vi "Top Level FPGA_w8LED.vi"() -> ()   [LabVIEW 2012]
uses:
  <vilib>/Platform/TimedLoop/XDataNode/timing_clust.ctl
  <vilib>/Platform/TimedLoop/XDataNode/nitl_modes.ctl
  <vilib>/Platform/TimedLoop/XDataNode/wakeup.ctl
  <vilib>/rvi/DataTransferAndStorage/Container/Common/niFpgaContainerMetaDataKey.ctl
  <vilib>/rvi/DataTransferAndStorage/Container/Common/niFpgaContainerState.ctl
  <vilib>/rvi/DataTransferAndStorage/Container/Common/niFpgaDataTypeControl.ctl
  <vilib>/rvi/DataTransferAndStorage/Container/Common/niFpgaContainerImplementationControl.ctl
  <vilib>/rvi/DataTransferAndStorage/Container/Common/niFpgaContainerArbitrationOptionsControl.ctl
  <vilib>/rvi/DataTransferAndStorage/Container/Common/niFpgaTransferTypeControl.ctl
  <vilib>/rvi/DataTransferAndStorage/Container/Common/niFpgaContainerInitializationParameters.ctl
  <vilib>/rvi/Memory/Memory_Types/niFpgaMemoryInterfaceConfiguration.ctl
  <vilib>/rvi/FIFO/Fifo_Types/niFpgaFifoControlLogicControl.ctl
  <vilib>/rvi/eio/common/nirviEmuTemplateMethod_errors.vi
  <vilib>/rvi/FIFO/Fifo_Resource/nirvififoEmulationSetSize.vi
  <vilib>/rvi/DataTransferAndStorage/Container/Common/niFpgaContainerGetUniqueNameForEmu.vi
  <vilib>/rvi/Emulation/niFpgaSctlEmulationRegisterWithScheduler.vi
  <vilib>/rvi/Emulation/niFpgaSctlEmulationScheduler.vi
  <vilib>/rvi/DataTransferAndStorage/Container/Common/niFpgaContainerSetEmuInfo.vi
  <vilib>/rvi/eio/common/nirviEmuReportErrorAndStop.vi
  <vilib>/rvi/Emulation/niFpgaSctlEmulationFifoFullMgr.vi
  <vilib>/rvi/errors/niFpgaSetErrorForExecOnDevCompSimple.vi
  <vilib>/rvi/Memory/Memory_Emulation/nirvimemoryEmulationManagerCache_GetValue.vi
  <vilib>/rvi/Memory/Memory_Emulation/niFpgaMemoryEmulationValidateCache.vi
  <vilib>/rvi/Memory/Memory_Emulation/nirvimemoryEmulationManagerCache_InsertValue.vi
  <vilib>/rvi/Memory/Memory_Emulation/nirvimemoryEmulationManagerCache_SetValue.vi
  <vilib>/rvi/Emulation/niFpgaSctlEmulationResourceMgr.vi
  <vilib>/rvi/Memory/Memory_Emulation/niFpgaMemoryEmulationCacheClearOnFirstRun.vi
  <vilib>/rvi/Memory/Memory_Emulation/nirvimemoryEmulationManagerCache_MakeExclusive.vi
  <vilib>/rvi/Memory/Memory_Emulation/nirvimemoryEmulationManagerCache_ReleaseExclusive.vi
  <vilib>/Utility/error.llb/Clear Errors.vi
  <vilib>/eio/EIONode/EIONode.xnode
  <vilib>/Platform/TimedLoop/XDataNode/XDataNode.xnode
  <vilib>/rvi/DataTransferAndStorage/Container/XNode/niFpgaContainer.xnode
  <vilib>/rvi/FIFO/Fifo_Resource/nirvififoEmulationClear.vi
  <vilib>/rvi/LocalResourceManager/LocalResourceManager.xnode
  <vilib>/rvi/FIFO/Fifo_Resource/nirvififoEmulationRead.vi
  <vilib>/rvi/DataTransferAndStorage/Register/Emulation/niFpgaRegisterEmulation.vi
  <vilib>/rvi/Memory/Memory_Emulation/nirvimemoryEmulation.vi
  <vilib>/rvi/FIFO/Fifo_Resource/nirvififoEmulationWrite.vi
  <vilib>/Platform/TimedLoop/XDataNode/XDNodeRunTimeDep.lvlib
panel:
  out "IO Module\\ADC Error A":bool
  out "IO Module\\ADC Error B":bool
  out "IO Module\\Pll Unlocked":bool
  in  "Record Size only data":u32=95
  out "DMA FIFO Timed Out?":bool
  in  "circular buffer length":u32=1000
  in  "location":i16(ring) items=["Purdue", "NIKHEF", "Zurich", "???"]
  in  "Trigger 0":i16=4000
  in  "Trigger 1":i16=4000
  in  "Trigger 2":i16=4000
  in  "Trigger 3":i16=4000
  in  "Trigger 4":i16=4000
  in  "Trigger 5":i16=4000
  in  "Trigger 6":i16=4000
  in  "Trigger 7":i16=4000
  in  "# of pretrigger":u32=20
  in  "initial value":u64
  in  "channel 0 on/off":bool
  in  "channel 2 on/off":bool
  in  "channel 1 on/off":bool
  in  "channel 3 on/off":bool
  in  "channel 4 on/off":bool
  in  "channel 5 on/off":bool
  in  "channel 6 on/off":bool
  in  "channel 7 on/off":bool
  in  "Testpulse duration (20 ns ticks)":u32=1
  in  "Testpulse Separation (20 ns ticks)":u32=500
  in  "Testpulse Time Delay (20 ns ticks)":u32=15
  out "Timestamp":u64
  in  "Testpulser On/Off":bool
  out "Init Done":bool
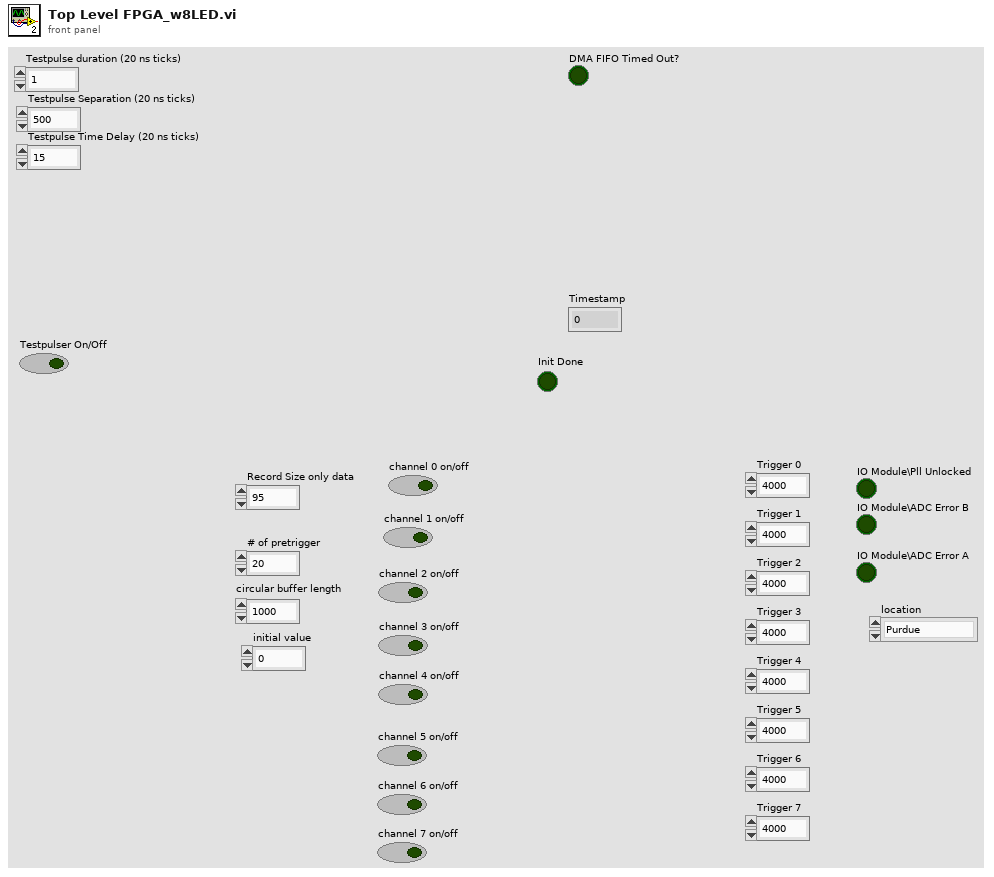
[diagram p1: front panel]
types:
  T1 = typedef "XDNodeRunTimeDep.lvlib/timing_clust.ctl" = cluster{"Expected End [f-1]":u64, "Actual End [f-1]":u64, "Finished Late? [f-1]":bool, "Expected End [i-1]":u64, "Actual End [i-1]":u64, "Finished Late? [i-1]":bool, "Expected Start [i]":u64, "Actual Start [i]":u64, "Expected Start [f]":u64, "Actual Start [f]":u64, "Source Name":string, "Structure Name":string, "Period":i64, "Deadline":i64, "Offset":i64, "Start":i64, "Priority":i32, "Timeout":i32, "Mode":T2, "Wakeup Reason":T3, "Error":errorcluster, "Source Type":string, "Secondary Source Type":string, "Global End Time":u64, "Global Start Time":u64, "Frame Duration":u64, "Iteration Duration":u64, "Assigned CPU":i32, "I/O Scan Engine Mode":u32}
  T2 = typedef "XDNodeRunTimeDep.lvlib/nitl_modes.ctl" = enum32{"No Change", "Process missed periods, maintain original phase", "Discard missed periods, maintain original phase", "Process missed periods, ignore original phase", "Discard missed periods, ignore original phase"}
  T3 = typedef "XDNodeRunTimeDep.lvlib/wakeup.ctl" = enum32{"Normal", "Aborted", "Asynchronous wakeup", "Timing source error", "Timed loop error", "Timeout"}
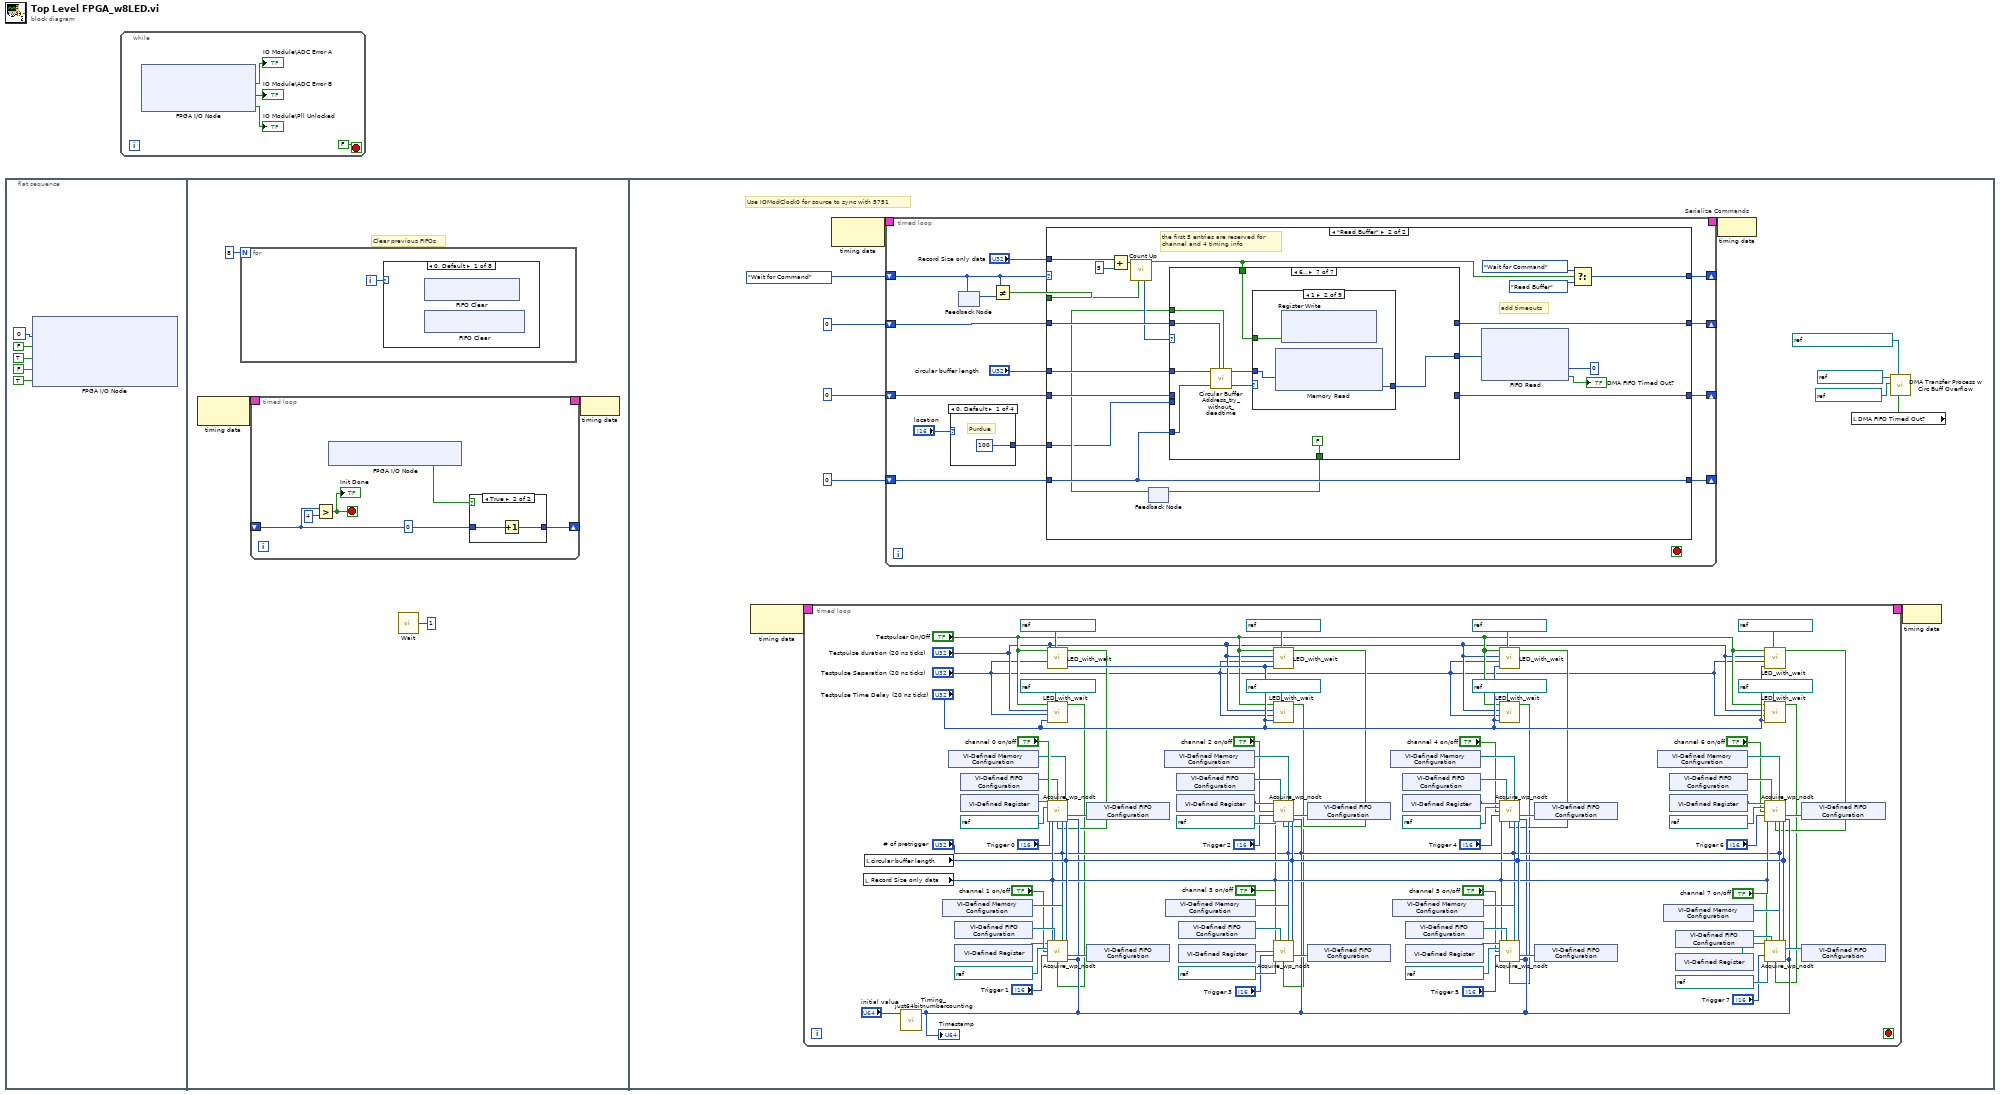
[diagram p0: block diagram]
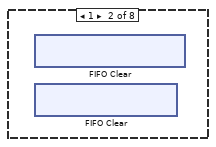
[diagram p2: hidden frame]
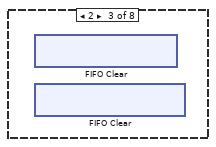
[diagram p3: hidden frame]
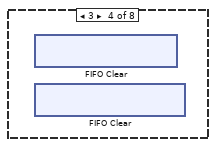
[diagram p4: hidden frame]
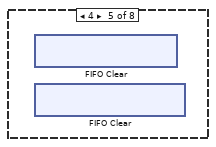
[diagram p5: hidden frame]
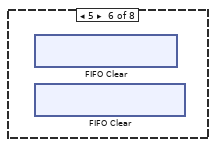
[diagram p6: hidden frame]
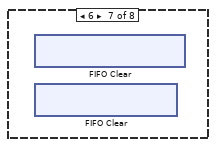
[diagram p7: hidden frame]
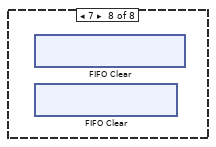
[diagram p8: hidden frame]
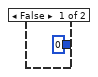
[diagram p9: hidden frame]
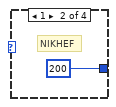
[diagram p10: hidden frame]
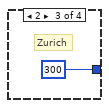
[diagram p11: hidden frame]
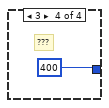
[diagram p12: hidden frame]
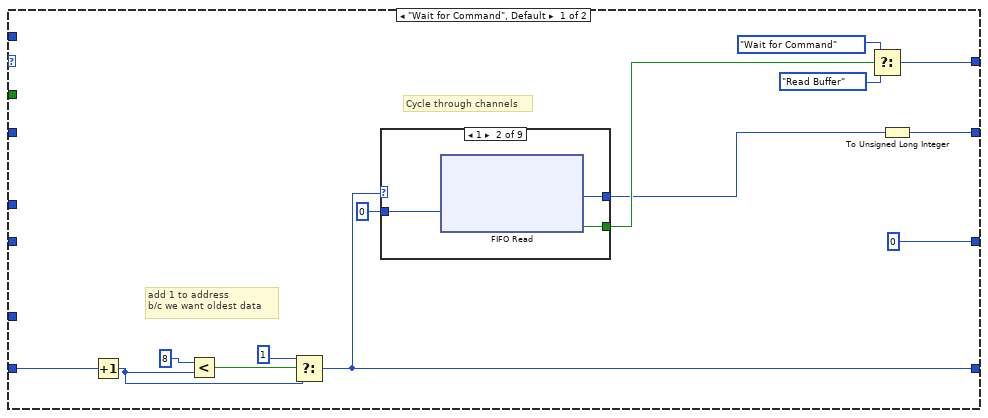
[diagram p13: hidden frame]
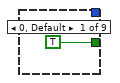
[diagram p14: hidden frame]
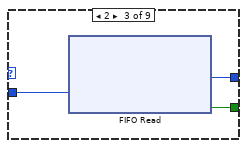
[diagram p15: hidden frame]
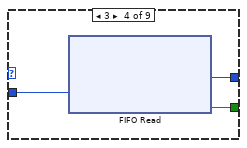
[diagram p16: hidden frame]
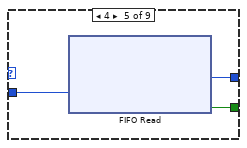
[diagram p17: hidden frame]
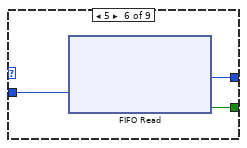
[diagram p18: hidden frame]
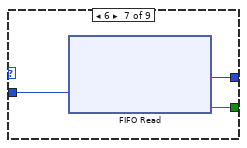
[diagram p19: hidden frame]
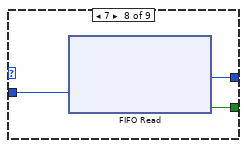
[diagram p20: hidden frame]
diagram:
  n1 = flat-sequence {
    frame #0 {
      n2 = xnode "FPGA I/O Node"("IO Module\\Sample Clock Select"=u8 0 ("IO Module\\Sample Clock Select"), "IO Module\\Force Initialization"=FALSE ("IO Module\\Force Initialization"), "IO Module\\Force Initialization"=TRUE ("IO Module\\Force Initialization"), "IO Module\\Force Initialization"=FALSE ("IO Module\\Force Initialization"), "IO Module\\Digital Output Enable"=TRUE ("IO Module\\Digital Output Enable")) -> ()  [unwired: 5 in, 5 out]
    }
    frame #1 {
      # "Clear previous FIFOs"
      n3 = node-c288() -> (w10:T1)  [unwired: 1 in]
      n4 = for {
        N: 8 -> [_]
        i -> [w11]
        n5 = case shown="0, Default" w11 {
          frame 0, Default {
            n6 = xnode ("FIFO Clear")() -> ()  [unwired: 1 in, 1 out]
            n7 = xnode ("FIFO Clear")() -> ()  [unwired: 1 in, 1 out]
          }
          frame 1 {
            n8 = xnode ("FIFO Clear")() -> ()  [unwired: 1 in, 1 out]
            n9 = xnode ("FIFO Clear")() -> ()  [unwired: 1 in, 1 out]
          }
          frame 2 {
            n10 = xnode ("FIFO Clear")() -> ()  [unwired: 1 in, 1 out]
            n11 = xnode ("FIFO Clear")() -> ()  [unwired: 1 in, 1 out]
          }
          frame 3 {
            n12 = xnode ("FIFO Clear")() -> ()  [unwired: 1 in, 1 out]
            n13 = xnode ("FIFO Clear")() -> ()  [unwired: 1 in, 1 out]
          }
          frame 4 {
            n14 = xnode ("FIFO Clear")() -> ()  [unwired: 1 in, 1 out]
            n15 = xnode ("FIFO Clear")() -> ()  [unwired: 1 in, 1 out]
          }
          frame 5 {
            n16 = xnode ("FIFO Clear")() -> ()  [unwired: 1 in, 1 out]
            n17 = xnode ("FIFO Clear")() -> ()  [unwired: 1 in, 1 out]
          }
          frame 6 {
            n18 = xnode ("FIFO Clear")() -> ()  [unwired: 1 in, 1 out]
            n19 = xnode ("FIFO Clear")() -> ()  [unwired: 1 in, 1 out]
          }
          frame 7 {
            n20 = xnode ("FIFO Clear")() -> ()  [unwired: 1 in, 1 out]
            n21 = xnode ("FIFO Clear")() -> ()  [unwired: 1 in, 1 out]
          }
        }
      }
      n22 = timed-loop {
        shift-right: [w15] -> _
        shift-left: u16 0 -> [w14]
        timing: w10 -> [_]
        timing-out: [_] -> w9
        stop <- w12 stop-if-true
        n23 = Greater?(x=w14, y=u16 4) -> (0:w12:bool)
        "Init Done" <- w12
        n24 = xnode "FPGA I/O Node"() -> ("IO Module\\Initialization Done"=w16:bool)  [unwired: 1 in, 1 out]
        n25 = case shown="True" w16 {
          tunnel: [u16 0 w19] -> w15
          tunnel: w14 -> [_ w18]
          frame False {
          }
          frame True {
            n26 = Increment(x=w18) -> (x+1=w19:u16)
          }
        }
      }
      n27 = call "Wait"("Count(mSec)"=u32 1) -> ()  [unwired: 1 out]
      n28 = node-c288(w9) -> ()
    }
    frame #2 {
      # "Use IOModClock0 for source to sync with 5751"
      n29 = node-c288() -> (w33:T1)  [unwired: 1 in]
      n30 = timed-loop {
        timing: w33 -> [_]
        timing-out: [_] -> w32
        stop <- _ stop-if-true
        n31 = local read "Record Size only data"() -> (w76:u32)
        n32 = local read "circular buffer length"() -> (w77:u32)
        n33 = call "Timing_just64bitnumbercounting.vi"("initial value"="initial value") -> ("x+1"=w47:u64)  [unwired: 10 in]
        "Timestamp" <- w47
        n34 = xnode "VI-Defined Memory Configuration"() -> ("Memory Out"=w116:refnum<k21>)
        n35 = xnode "VI-Defined Memory Configuration"() -> ("Memory Out"=w78:refnum<k21>)
        n36 = xnode "VI-Defined FIFO Configuration"() -> ("FIFO Out"=w115:refnum<k21>)
        n37 = xnode "VI-Defined Register"() -> ("Register Out"=w72:refnum<k21>)
        n38 = xnode "VI-Defined FIFO Configuration"() -> ("FIFO Out"=w79:refnum<k21>)
        n39 = xnode "VI-Defined Register"() -> ("Register Out"=w73:refnum<k21>)
        n40 = call "LED_with_wait.vi"("FPGA I/O In"=refnum<k21> "IO Module\\D0 0", "Testpulse Time Delay (20 ns ticks)"="Testpulse Time Delay (20 ns ticks)", "Testpulse Separation (20 ns ticks)"="Testpulse Separation (20 ns ticks)", "Testpulse duration (20 ns ticks)"="Testpulse duration (20 ns ticks)", "Testpulser On/Off"="Testpulser On/Off") -> ("Is Test Pulse?"=w46:bool)  [unwired: 5 in, 1 out]
        n41 = call "LED_with_wait.vi"("FPGA I/O In"=refnum<k21> "IO Module\\D0 1", "Testpulse Time Delay (20 ns ticks)"="Testpulse Time Delay (20 ns ticks)", "Testpulse Separation (20 ns ticks)"="Testpulse Separation (20 ns ticks)", "Testpulse duration (20 ns ticks)"="Testpulse duration (20 ns ticks)", "Testpulser On/Off"="Testpulser On/Off") -> ("Is Test Pulse?"=w45:bool)  [unwired: 5 in, 1 out]
        n42 = xnode "VI-Defined FIFO Configuration"() -> ("FIFO Out"=w64:refnum<k21>)
        n43 = call "Acquire_wp_nodt.vi"("Ch Armed Reg"=w73, "Command FIFO"=w79, "Circular Buffer Mem"=w78, "circular buffer length"=w77, "FPGA I/O In"=refnum<k21> "IO Module\\AI A0", "channel on/off"="channel 0 on/off", "Trigger"="Trigger 0", "Timing FIFO"=w64, "Samples to Acquire"=w76, "Is Test Pulse?"=w46, "# of pretrigger"="# of pretrigger", "timing"=w47) -> ()  [unwired: 4 in]
        n44 = xnode "VI-Defined FIFO Configuration"() -> ("FIFO Out"=w57:refnum<k21>)
        n45 = call "Acquire_wp_nodt.vi"("Ch Armed Reg"=w72, "Command FIFO"=w115, "Circular Buffer Mem"=w116, "circular buffer length"=w77, "FPGA I/O In"=refnum<k21> "IO Module\\AI A1", "channel on/off"="channel 1 on/off", "Trigger"="Trigger 1", "Timing FIFO"=w57, "Samples to Acquire"=w76, "Is Test Pulse?"=w45, "# of pretrigger"="# of pretrigger", "timing"=w47) -> ()  [unwired: 4 in]
        n46 = xnode "VI-Defined Memory Configuration"() -> ("Memory Out"=w112:refnum<k21>)
        n47 = xnode "VI-Defined Memory Configuration"() -> ("Memory Out"=w113:refnum<k21>)
        n48 = xnode "VI-Defined FIFO Configuration"() -> ("FIFO Out"=w111:refnum<k21>)
        n49 = xnode "VI-Defined Register"() -> ("Register Out"=w99:refnum<k21>)
        n50 = xnode "VI-Defined FIFO Configuration"() -> ("FIFO Out"=w114:refnum<k21>)
        n51 = xnode "VI-Defined Register"() -> ("Register Out"=w101:refnum<k21>)
        n52 = call "LED_with_wait.vi"("FPGA I/O In"=refnum<k21> "IO Module\\D0 2", "Testpulse Time Delay (20 ns ticks)"="Testpulse Time Delay (20 ns ticks)", "Testpulse Separation (20 ns ticks)"="Testpulse Separation (20 ns ticks)", "Testpulse duration (20 ns ticks)"="Testpulse duration (20 ns ticks)", "Testpulser On/Off"="Testpulser On/Off") -> ("Is Test Pulse?"=w44:bool)  [unwired: 5 in, 1 out]
        n53 = call "LED_with_wait.vi"("FPGA I/O In"=refnum<k21> "IO Module\\D0 3", "Testpulse Time Delay (20 ns ticks)"="Testpulse Time Delay (20 ns ticks)", "Testpulse Separation (20 ns ticks)"="Testpulse Separation (20 ns ticks)", "Testpulse duration (20 ns ticks)"="Testpulse duration (20 ns ticks)", "Testpulser On/Off"="Testpulser On/Off") -> ("Is Test Pulse?"=w43:bool)  [unwired: 5 in, 1 out]
        n54 = xnode "VI-Defined FIFO Configuration"() -> ("FIFO Out"=w63:refnum<k21>)
        n55 = call "Acquire_wp_nodt.vi"("Ch Armed Reg"=w99, "Command FIFO"=w111, "Circular Buffer Mem"=w112, "circular buffer length"=w77, "FPGA I/O In"=refnum<k21> "IO Module\\AI A2", "channel on/off"="channel 2 on/off", "Trigger"="Trigger 2", "Timing FIFO"=w63, "Samples to Acquire"=w76, "Is Test Pulse?"=w44, "# of pretrigger"="# of pretrigger", "timing"=w47) -> ()  [unwired: 4 in]
        n56 = xnode "VI-Defined FIFO Configuration"() -> ("FIFO Out"=w58:refnum<k21>)
        n57 = call "Acquire_wp_nodt.vi"("Ch Armed Reg"=w101, "Command FIFO"=w114, "Circular Buffer Mem"=w113, "circular buffer length"=w77, "FPGA I/O In"=refnum<k21> "IO Module\\AI A3", "channel on/off"="channel 3 on/off", "Trigger"="Trigger 3", "Timing FIFO"=w58, "Samples to Acquire"=w76, "Is Test Pulse?"=w43, "# of pretrigger"="# of pretrigger", "timing"=w47) -> ()  [unwired: 4 in]
        n58 = xnode "VI-Defined Memory Configuration"() -> ("Memory Out"=w104:refnum<k21>)
        n59 = xnode "VI-Defined Memory Configuration"() -> ("Memory Out"=w105:refnum<k21>)
        n60 = xnode "VI-Defined FIFO Configuration"() -> ("FIFO Out"=w103:refnum<k21>)
        n61 = xnode "VI-Defined Register"() -> ("Register Out"=w93:refnum<k21>)
        n62 = xnode "VI-Defined FIFO Configuration"() -> ("FIFO Out"=w106:refnum<k21>)
        n63 = xnode "VI-Defined Register"() -> ("Register Out"=w97:refnum<k21>)
        n64 = call "LED_with_wait.vi"("FPGA I/O In"=refnum<k21> "IO Module\\D0 4", "Testpulse Time Delay (20 ns ticks)"="Testpulse Time Delay (20 ns ticks)", "Testpulse Separation (20 ns ticks)"="Testpulse Separation (20 ns ticks)", "Testpulse duration (20 ns ticks)"="Testpulse duration (20 ns ticks)", "Testpulser On/Off"="Testpulser On/Off") -> ("Is Test Pulse?"=w42:bool)  [unwired: 5 in, 1 out]
        n65 = call "LED_with_wait.vi"("FPGA I/O In"=refnum<k21> "IO Module\\D0 5", "Testpulse Time Delay (20 ns ticks)"="Testpulse Time Delay (20 ns ticks)", "Testpulse Separation (20 ns ticks)"="Testpulse Separation (20 ns ticks)", "Testpulse duration (20 ns ticks)"="Testpulse duration (20 ns ticks)", "Testpulser On/Off"="Testpulser On/Off") -> ("Is Test Pulse?"=w41:bool)  [unwired: 5 in, 1 out]
        n66 = xnode "VI-Defined FIFO Configuration"() -> ("FIFO Out"=w62:refnum<k21>)
        n67 = call "Acquire_wp_nodt.vi"("Ch Armed Reg"=w93, "Command FIFO"=w103, "Circular Buffer Mem"=w104, "circular buffer length"=w77, "FPGA I/O In"=refnum<k21> "IO Module\\AI A4", "channel on/off"="channel 4 on/off", "Trigger"="Trigger 4", "Timing FIFO"=w62, "Samples to Acquire"=w76, "Is Test Pulse?"=w42, "# of pretrigger"="# of pretrigger", "timing"=w47) -> ()  [unwired: 4 in]
        n68 = xnode "VI-Defined FIFO Configuration"() -> ("FIFO Out"=w59:refnum<k21>)
        n69 = call "Acquire_wp_nodt.vi"("Ch Armed Reg"=w97, "Command FIFO"=w106, "Circular Buffer Mem"=w105, "circular buffer length"=w77, "FPGA I/O In"=refnum<k21> "IO Module\\AI A5", "channel on/off"="channel 5 on/off", "Trigger"="Trigger 5", "Timing FIFO"=w59, "Samples to Acquire"=w76, "Is Test Pulse?"=w41, "# of pretrigger"="# of pretrigger", "timing"=w47) -> ()  [unwired: 4 in]
        n70 = xnode "VI-Defined Memory Configuration"() -> ("Memory Out"=w109:refnum<k21>)
        n71 = xnode "VI-Defined Memory Configuration"() -> ("Memory Out"=w108:refnum<k21>)
        n72 = xnode "VI-Defined FIFO Configuration"() -> ("FIFO Out"=w110:refnum<k21>)
        n73 = xnode "VI-Defined Register"() -> ("Register Out"=w95:refnum<k21>)
        n74 = xnode "VI-Defined FIFO Configuration"() -> ("FIFO Out"=w107:refnum<k21>)
        n75 = xnode "VI-Defined Register"() -> ("Register Out"=w91:refnum<k21>)
        n76 = call "LED_with_wait.vi"("FPGA I/O In"=refnum<k21> "IO Module\\D0 6", "Testpulse Time Delay (20 ns ticks)"="Testpulse Time Delay (20 ns ticks)", "Testpulse Separation (20 ns ticks)"="Testpulse Separation (20 ns ticks)", "Testpulse duration (20 ns ticks)"="Testpulse duration (20 ns ticks)", "Testpulser On/Off"="Testpulser On/Off") -> ("Is Test Pulse?"=w40:bool)  [unwired: 5 in, 1 out]
        n77 = call "LED_with_wait.vi"("FPGA I/O In"=refnum<k21> "IO Module\\D0 7", "Testpulse Time Delay (20 ns ticks)"="Testpulse Time Delay (20 ns ticks)", "Testpulse Separation (20 ns ticks)"="Testpulse Separation (20 ns ticks)", "Testpulse duration (20 ns ticks)"="Testpulse duration (20 ns ticks)", "Testpulser On/Off"="Testpulser On/Off") -> ("Is Test Pulse?"=w39:bool)  [unwired: 5 in, 1 out]
        n78 = xnode "VI-Defined FIFO Configuration"() -> ("FIFO Out"=w61:refnum<k21>)
        n79 = call "Acquire_wp_nodt.vi"("Ch Armed Reg"=w95, "Command FIFO"=w110, "Circular Buffer Mem"=w109, "circular buffer length"=w77, "FPGA I/O In"=refnum<k21> "IO Module\\AI A6", "channel on/off"="channel 6 on/off", "Trigger"="Trigger 6", "Timing FIFO"=w61, "Samples to Acquire"=w76, "Is Test Pulse?"=w40, "# of pretrigger"="# of pretrigger", "timing"=w47) -> ()  [unwired: 4 in]
        n80 = xnode "VI-Defined FIFO Configuration"() -> ("FIFO Out"=w60:refnum<k21>)
        n81 = call "Acquire_wp_nodt.vi"("Ch Armed Reg"=w91, "Command FIFO"=w107, "Circular Buffer Mem"=w108, "circular buffer length"=w77, "FPGA I/O In"=refnum<k21> "IO Module\\AI A7", "channel on/off"="channel 7 on/off", "Trigger"="Trigger 7", "Timing FIFO"=w60, "Samples to Acquire"=w76, "Is Test Pulse?"=w39, "# of pretrigger"="# of pretrigger", "timing"=w47) -> ()  [unwired: 4 in]
      }
      n82 = node-c288() -> (w35:T1)  [unwired: 1 in]
      n83 = timed-loop "Serialize Commands" {
        timing: w35 -> [_]
        timing-out: [_] -> w34
        shift-right: [w897] -> _
        shift-left: enum16{"Wait for Command", "Read Buffer"}."Wait for Command" -> [w895]
        shift-right: [w901] -> _
        shift-left: u32 0 ("Element") -> [w900]
        shift-right: [w899] -> _
        shift-left: u8 0 ("t") -> [w898]
        shift-right: [w892] -> _
        shift-left: u64 0 ("Element") -> [w891]
        stop <- _ stop-if-true
        n84 = case shown="0, Default" "location" {
          tunnel: [i16 100 i16 200 i16 300 i16 400] -> w889
          frame 0, Default {
            # "Purdue"
          }
          frame 1 {
            # "NIKHEF"
          }
          frame 2 {
            # "Zurich"
          }
          frame 3 {
            # "???"
          }
        }
        n85 = feedback-in #1(w895) -> ()
        n86 = feedback #1() -> (w896:enum16{"Wait for Command", "Read Buffer"})  [unwired: 1 in]
        n87 = Not Equal?(x=w895, y=w896) -> (x != y?=w893:bool)
        n88 = case shown="\"Read Buffer\"" w895 {
          tunnel: "Record Size only data" -> [_ w955]
          tunnel: [w909 w965] -> w899
          tunnel: w898 -> [w911 w965]
          tunnel: [w912 w950] -> w901
          tunnel: w900 -> [_ w964]
          tunnel: [w915 w966] -> w897
          tunnel: "circular buffer length" -> [_ w963]
          tunnel: w893 -> [_ w957]
          tunnel: [u64 0 ("Element") w952] -> w892
          tunnel: w891 -> [_ w951]
          tunnel: w889 -> [_ w946]
          frame "Wait for Command", Default {
            # "add 1 to address\nb/c we want oldest data"
            # "Cycle through channels"
            n89 = Increment(x=w911) -> (x+1=w910:u8)
            n90 = Less?(x=u8 8, y=w910) -> (x < y?=w919:bool)
            n91 = Select(t=u8 1, s=w919, f=w910) -> (s? t:f=w909:u8)
            n92 = case shown="1" w909 {
              tunnel: [TRUE ("Timed Out?") w924 w925 w928 w931 w934 w937 w940 w943] -> w916
              tunnel: 0 ("Timeout") -> [_ w923 w927 w930 w933 w936 w939 w942 w945]
              tunnel: [_ w922 w926 w929 w932 w935 w938 w941 w944] -> w908
              frame 0, Default {
              }
              frame 1 {
                n93 = xnode ("FIFO Read")("Timeout"=w923) -> ("Element"=w922:i16, "Timed Out?"=w924:bool)  [unwired: 1 in, 1 out]
              }
              frame 2 {
                n94 = xnode ("FIFO Read")("Timeout"=w927) -> ("Element"=w926:i16, "Timed Out?"=w925:bool)  [unwired: 1 in, 1 out]
              }
              frame 3 {
                n95 = xnode ("FIFO Read")("Timeout"=w930) -> ("Element"=w929:i16, "Timed Out?"=w928:bool)  [unwired: 1 in, 1 out]
              }
              frame 4 {
                n96 = xnode ("FIFO Read")("Timeout"=w933) -> ("Element"=w932:i16, "Timed Out?"=w931:bool)  [unwired: 1 in, 1 out]
              }
              frame 5 {
                n97 = xnode ("FIFO Read")("Timeout"=w936) -> ("Element"=w935:i16, "Timed Out?"=w934:bool)  [unwired: 1 in, 1 out]
              }
              frame 6 {
                n98 = xnode ("FIFO Read")("Timeout"=w939) -> ("Element"=w938:i16, "Timed Out?"=w937:bool)  [unwired: 1 in, 1 out]
              }
              frame 7 {
                n99 = xnode ("FIFO Read")("Timeout"=w942) -> ("Element"=w941:i16, "Timed Out?"=w940:bool)  [unwired: 1 in, 1 out]
              }
              frame 8 {
                n100 = xnode ("FIFO Read")("Timeout"=w945) -> ("Element"=w944:i16, "Timed Out?"=w943:bool)  [unwired: 1 in, 1 out]
              }
            }
            n101 = Select(t=enum16{"Wait for Command", "Read Buffer"}."Wait for Command", s=w916, f=enum16{"Wait for Command", "Read Buffer"}."Read Buffer") -> (s? t:f=w915:enum16{"Wait for Command", "Read Buffer"})
            n102 = To Unsigned Long Integer(number=w908) -> (unsigned 32bit integer=w912:u32)
          }
          frame "Read Buffer" {
            # "the first 5 entries are reserved for channel and 4 timing info"
            # "add timeouts"
            n103 = Add(x=w955, y=u32 5) -> (x+y=w953:u32)
            n104 = call "Count Up.vi"("Reset?"=w957, "goal"=w953) -> ("Count Met"=w959:bool, "count"=w956:u32)  [unwired: 8 in]
            n105 = feedback #2() -> (w949:bool)  [unwired: 1 in]
            n106 = case shown="6.." w956 {
              tunnel: w965 -> [_ w975 w982 _ _ _ w1021]
              tunnel: w964 -> [_ w979 w984 w1005 w1011 w1017 w1028]
              tunnel: w963 -> [_ _ _ _ _ _ w1027]
              tunnel: w959 -> [_ _ _ _ _ _ w1026]
              tunnel: [i16 0 ("Data") w976 w986 w1003 w1009 w1015 w1022] -> w958
              tunnel: w949 -> [_ _ _ _ _ _ w1024]
              tunnel: [u64 0 ("Element") _ w983 w1006 w1012 w1018 _] -> w952
              tunnel: w951 -> [_ _ _ w1006 w1012 w1018 _]
              tunnel: [u32 0 ("Element") w979 w984 w1005 w1011 w1017 _] -> w950
              tunnel: [FALSE FALSE FALSE FALSE FALSE TRUE FALSE] -> w948
              tunnel: w946 -> [_ w971 _ _ _ _ _]
              frame 0, Default {
              }
              frame 1 {
                w977 = u16 0 items=["Header Information", "Particle Pulse", "Test Pulse"] ("Pulse Type")
                n107 = Decrement(x=w975) -> (x-1=w974:u8)
                n108 = To Word Integer(number=w974) -> (16bit integer=w973:i16)
                n109 = Add(x=w971, y=w973) -> (x+y=w972:i16)
                n110 = call "bitmanip.vi"("Pulse Type"=w977, "Integer to be written"=w972) -> ("Integer Written"=w976:i16)  [unwired: 2 in]
              }
              frame 2 {
                # "reads out the lsb of the timing information"
                n111 = case shown="1" w982 {
                  tunnel: [_ w987 w989 w991 w993 w995 w997 w999 w1001] -> w983
                  frame Default {
                  }
                  frame 1 {
                    n112 = xnode ("FIFO Read")("Timeout"=0) -> ("Element"=w987:u64)  [unwired: 1 in, 2 out]
                  }
                  frame 2 {
                    n113 = xnode ("FIFO Read")("Timeout"=0) -> ("Element"=w989:u64)  [unwired: 1 in, 2 out]
                  }
                  frame 3 {
                    n114 = xnode ("FIFO Read")("Timeout"=0) -> ("Element"=w991:u64)  [unwired: 1 in, 2 out]
                  }
                  frame 4 {
                    n115 = xnode ("FIFO Read")("Timeout"=0) -> ("Element"=w993:u64)  [unwired: 1 in, 2 out]
                  }
                  frame 5 {
                    n116 = xnode ("FIFO Read")("Timeout"=0) -> ("Element"=w995:u64)  [unwired: 1 in, 2 out]
                  }
                  frame 6 {
                    n117 = xnode ("FIFO Read")("Timeout"=0) -> ("Element"=w997:u64)  [unwired: 1 in, 2 out]
                  }
                  frame 7 {
                    n118 = xnode ("FIFO Read")("Timeout"=0) -> ("Element"=w999:u64)  [unwired: 1 in, 2 out]
                  }
                  frame 8 {
                    n119 = xnode ("FIFO Read")("Timeout"=0) -> ("Element"=w1001:u64)  [unwired: 1 in, 2 out]
                  }
                }
                n120 = Split Number(x=w983) -> (hi(x)=w981:u32)  [unwired: 1 out]
                n121 = Split Number(x=w981) -> (hi(x)=w980:u16)  [unwired: 1 out]
                n122 = To Word Integer(number=w980) -> (16bit integer=w986:i16)
              }
              frame 3 {
                n123 = Split Number(x=w1006) -> (hi(x)=w1008:u32)  [unwired: 1 out]
                n124 = Split Number(x=w1008) -> (lo(x)=w1007:u16)  [unwired: 1 out]
                n125 = To Word Integer(number=w1007) -> (16bit integer=w1003:i16)
              }
              frame 4 {
                n126 = Split Number(x=w1012) -> (lo(x)=w1014:u32)  [unwired: 1 out]
                n127 = Split Number(x=w1014) -> (hi(x)=w1013:u16)  [unwired: 1 out]
                n128 = To Word Integer(number=w1013) -> (16bit integer=w1009:i16)
              }
              frame 5 {
                n129 = Split Number(x=w1018) -> (lo(x)=w1020:u32)  [unwired: 1 out]
                n130 = Split Number(x=w1020) -> (lo(x)=w1019:u16)  [unwired: 1 out]
                n131 = To Word Integer(number=w1019) -> (16bit integer=w1015:i16)
              }
              frame 6.. {
                n132 = call "Circular Buffer Address_try_without_deadtime.vi"("Reset?"=w1024, "Starting Address"=w1028, "circular buffer length"=w1027) -> ("Address"=w1025:u32)  [unwired: 8 in]
                n133 = case shown="1" w1021 {
                  tunnel: w1025 -> [_ w1032 w1035 w1038 w1041 w1044 w1047 w1050 w1053]
                  tunnel: w1026 -> [_ w1031 w1034 w1037 w1040 w1043 w1046 w1049 w1052]
                  tunnel: [i16 0 w1030 w1033 w1036 w1039 w1042 w1045 w1048 w1051] -> w1022
                  frame Default {
                    # "Error"
                  }
                  frame 1 {
                    n134 = xnode ("Memory Read")("Address"=w1032) -> ("Data"=w1030:i16)  [unwired: 1 in, 1 out]
                    n135 = xnode ("Register Write")("Data"=w1031) -> ()  [unwired: 1 in, 1 out]
                  }
                  frame 2 {
                    n136 = xnode ("Memory Read")("Address"=w1035) -> ("Data"=w1033:i16)  [unwired: 1 in, 1 out]
                    n137 = xnode ("Register Write")("Data"=w1034) -> ()  [unwired: 1 in, 1 out]
                  }
                  frame 3 {
                    n138 = xnode ("Memory Read")("Address"=w1038) -> ("Data"=w1036:i16)  [unwired: 1 in, 1 out]
                    n139 = xnode ("Register Write")("Data"=w1037) -> ()  [unwired: 1 in, 1 out]
                  }
                  frame 4 {
                    n140 = xnode ("Memory Read")("Address"=w1041) -> ("Data"=w1039:i16)  [unwired: 1 in, 1 out]
                    n141 = xnode ("Register Write")("Data"=w1040) -> ()  [unwired: 1 in, 1 out]
                  }
                  frame 5 {
                    n142 = xnode ("Memory Read")("Address"=w1044) -> ("Data"=w1042:i16)  [unwired: 1 in, 1 out]
                    n143 = xnode ("Register Write")("Data"=w1043) -> ()  [unwired: 1 in, 1 out]
                  }
                  frame 6 {
                    n144 = xnode ("Memory Read")("Address"=w1047) -> ("Data"=w1045:i16)  [unwired: 1 in, 1 out]
                    n145 = xnode ("Register Write")("Data"=w1046) -> ()  [unwired: 1 in, 1 out]
                  }
                  frame 7 {
                    n146 = xnode ("Memory Read")("Address"=w1050) -> ("Data"=w1048:i16)  [unwired: 1 in, 1 out]
                    n147 = xnode ("Register Write")("Data"=w1049) -> ()  [unwired: 1 in, 1 out]
                  }
                  frame 8 {
                    n148 = xnode ("Memory Read")("Address"=w1053) -> ("Data"=w1051:i16)  [unwired: 1 in, 1 out]
                    n149 = xnode ("Register Write")("Data"=w1052) -> ()  [unwired: 1 in, 1 out]
                  }
                }
              }
            }
            n150 = feedback-in #2(w948) -> ()
            n151 = xnode ("FIFO Read")("Element"=w958, "Timeout"=0) -> ("Timed Out?"=→"DMA FIFO Timed Out?":bool)  [unwired: 1 in, 1 out]
            n152 = Select(t=enum16{"Wait for Command", "Read Buffer"}."Wait for Command", s=w959, f=enum16{"Wait for Command", "Read Buffer"}."Read Buffer") -> (s? t:f=w966:enum16{"Wait for Command", "Read Buffer"})
          }
        }
      }
      n153 = node-c288(w34) -> ()
      n154 = local read "DMA FIFO Timed Out?"() -> (w27:bool)
      n155 = call "DMA Transfer Process w Circ Buff Overflow.vi"("DMA Write Timed Out?"=w27, "Clock Domain"=refnum<k21> "40 MHz Onboard Clock", "Local"=refnum<k21> "To DMA FIFO", "DMA"=refnum<k21> "To Host FIFO") -> ()  [unwired: 8 in]
      n156 = node-c288(w32) -> ()
    }
  }
  n157 = while {
    stop <- FALSE stop-if-true
    n158 = xnode "FPGA I/O Node"() -> ("IO Module\\ADC Error A"=→"IO Module\\ADC Error A":bool, "IO Module\\ADC Error B"=→"IO Module\\ADC Error B":bool, "IO Module\\Pll Unlocked"=→"IO Module\\Pll Unlocked":bool)  [unwired: 3 in, 3 out]
  }
